vi "toggleShutter.vi"(7 "Error In":errorcluster) -> (0 "error out":errorcluster)   [LabVIEW 2014]
doc: "Newport Motion Controler\nThis program Toggle Shutter (open / close)\n\nAndré Romero - 2020\nandretec@ifsc.usp.br"
uses:
  Global Shutter.vi
panel:
  out "VISA Refnum out":refnum<visa-resource-name>
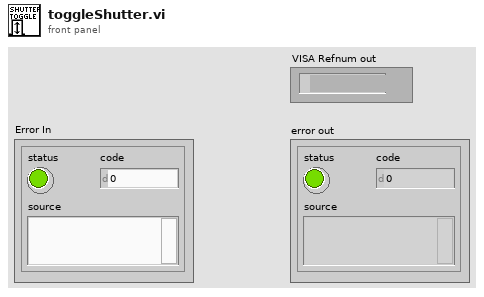
[diagram p1: front panel]
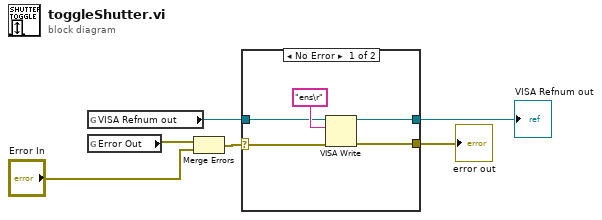
[diagram p0: block diagram]
diagram:
  n1 = global read "Global Shutter.vi" "VISA Refnum out"() -> (w4:refnum<visa-resource-name>)
  n2 = global read "Global Shutter.vi" "Error Out"() -> (w2:errorcluster)
  n3 = Merge Errors(w2, "Error In") -> (w3:errorcluster)
  n4 = case shown="No Error" w3 {
    selector: w3 -> [w7 w12]
    tunnel: [w11 w12] -> w6
    tunnel: [w10 w13] -> w5
    tunnel: w4 -> [w8 w13]
    frame No Error {
      n5 = VISA Write(VISA resource name=w8, write buffer="ens\r", error in (no error)=w7) -> (VISA resource name out=w10:refnum<visa-resource-name>, error out=w11:errorcluster)  [unwired: 1 out]
    }
    frame Error {
    }
  }
  "error out" <- w6
  "VISA Refnum out" <- w5
